vi "x_y(F.R).vi"(6 "Sensor 8":dbl, 7 "Array":dbl[](array[numeric]), 9 "Sensor 7":dbl, 10 "Sensor 6":dbl, 11 "Sensor 5":dbl) -> (1 "Sum(F.R)":dbl, 2 "y(F.R)":dbl, 3 "x(F.R)":dbl)   [LabVIEW 2019]
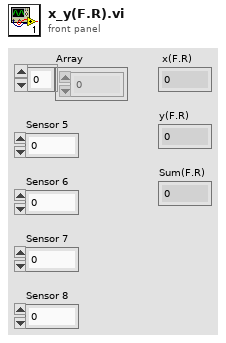
[diagram p1: front panel]
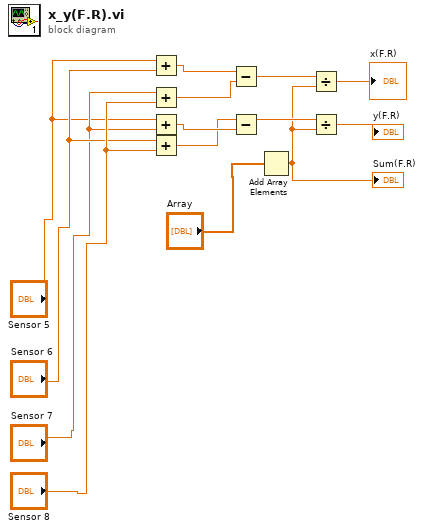
[diagram p0: block diagram]
diagram:
  n1 = Add(x="Sensor 5", y="Sensor 6") -> (x+y=w4:dbl)
  n2 = Add(x="Sensor 7", y="Sensor 8") -> (x+y=w3:dbl)
  n3 = Add(x="Sensor 5", y="Sensor 7") -> (x+y=w2:dbl)
  n4 = Add(x="Sensor 6", y="Sensor 8") -> (x+y=w1:dbl)
  n5 = Subtract(x=w4, y=w3) -> (x-y=w7:dbl)
  n6 = Subtract(x=w1, y=w2) -> (x-y=w8:dbl)
  n7 = Add Array Elements(numeric array="Array") -> (sum=w5:dbl)
  "Sum(F.R)" <- w5
  n8 = Divide(x=w7, y=w5) -> (x/y=→"x(F.R)":dbl)
  n9 = Divide(x=w8, y=w5) -> (x/y=→"y(F.R)":dbl)
